vi "Write Setting.vi"(8 "error in (no error)":errorcluster, 10 "Setting":bool, 11 "Update Boolean in":refnum<class "Update Boolean.lvclass">) -> (0 "error out":errorcluster, 3 "Update Boolean out":refnum<class "Update Boolean.lvclass">)   [LabVIEW 2014, in "Update Boolean.lvclass"]
uses:
  Update Boolean.lvclass
  Update Boolean.lvclass/Update Boolean.ctl
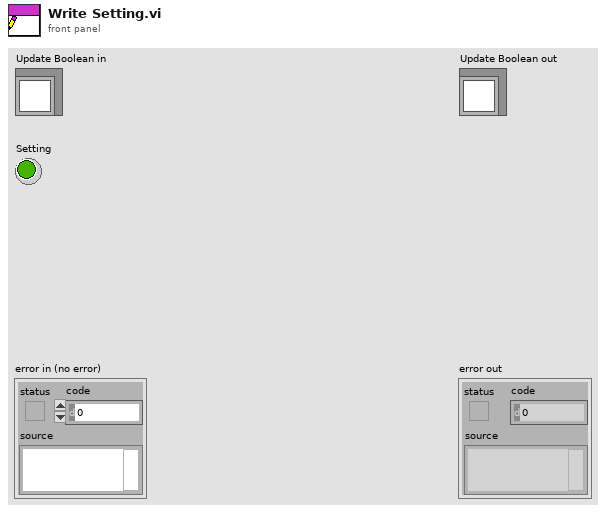
[diagram p1: front panel]
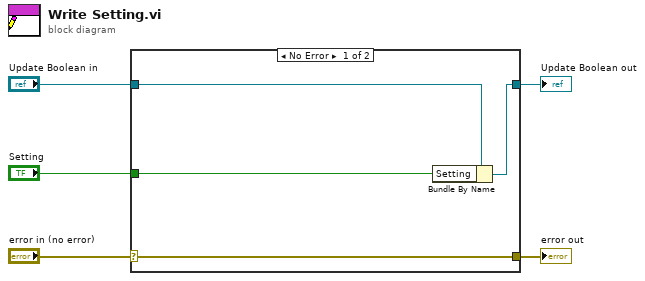
[diagram p0: block diagram]
diagram:
  n1 = case shown="No Error" "error in (no error)" {
    selector: "error in (no error)" -> [w9 w10]
    tunnel: [w9 w10] -> w4
    tunnel: [w7 w11] -> w2
    tunnel: "Update Boolean in" -> [w8 w11]
    tunnel: "Setting" -> [w6 _]
    frame No Error {
      n2 = Bundle By Name(cluster=w8, "Setting"=w6) -> (w7:refnum<class "Update Boolean.lvclass">)
    }
    frame Error {
    }
  }
  "error out" <- w4
  "Update Boolean out" <- w2
